vi "HALF_ADDER.vi"() -> ()   [LabVIEW 2020]
panel:
  out "CARRY":bool
  out "SUM":bool
  in  "B":bool
  in  "A":bool
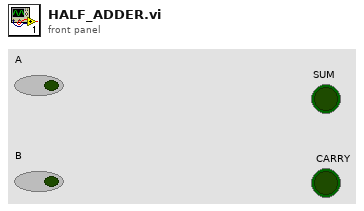
[diagram p1: front panel]
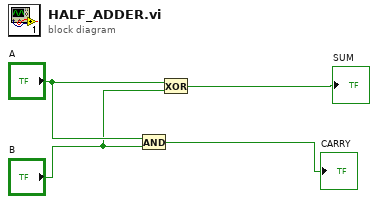
[diagram p0: block diagram]
diagram:
  n1 = And(x="A", y="B") -> (x .and. y?=→"CARRY":bool)
  n2 = Exclusive Or(1:"B", 2:"A") -> (0:→"SUM":bool)
